vi "Draw GUI running average centroid overlay.vi"(8 "error in":errorcluster, 10 "GUI_centroid overlay":T2={"CentroidX array"=[], "CentroidY array"=[], "CentroidX"=0.0, "CentroidY"=0.0, "# images to average"=1250067, "Overlay Size"={"xhair size"=0.0, "xhair size 2"=0.0}, "Color"=1250067, "Draw"=FALSE, "Thickness"=0}, 11 "Image in":T3) -> (0 "error out":errorcluster, 3 "image out":T3)   [LabVIEW 2020]
doc: "Draw Crosshair in image as per targetx and y and size\ninput:\n1. Draw crosshair cluster (Image in, Draw(boolean), size, target x, target y)\n2. Error in\noutput\n1.Error out"
uses:
  <vilib>/vision/Image Controls.llb/IMAQ Image.ctl
  Controls/GUI_running average centroid overlay.ctl
  General GUIs/Device GUIs/GUI_Cameras/Controls/Crosshair type def.ctl
  <vilib>/ptbypt/NI_PtbyPt.lvlib
panel:
  in  "Crosshair":T1={"Draw"=TRUE, "Target"={"x"=75.0, "y"=100.0}, "Size"={"x"=75.0, "y"=100.0}, "Angle"=1250067.0, "Color"=1250067, "Thickness"=20, "CrosshairLabel"=""} {"Thickness" max=0; "Angle" format="%#_13g"; "Size"."y" min=0.0 max=0.0; "Size"."x" min=0.0 max=0.0}
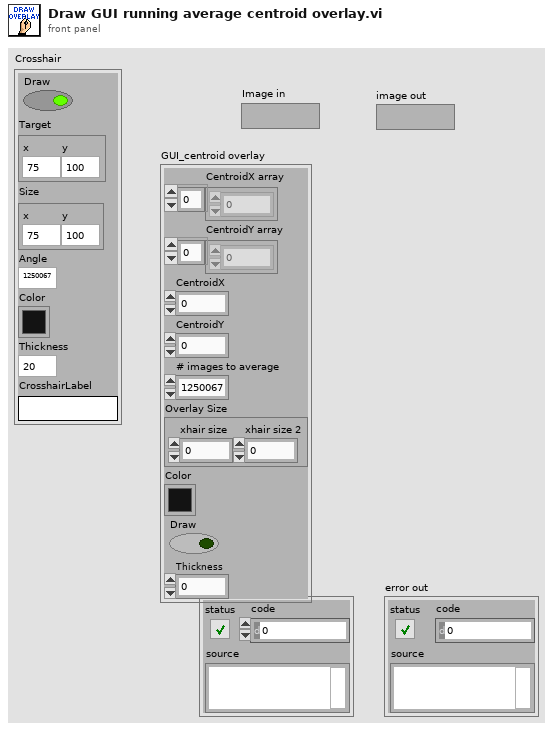
[diagram p1: front panel]
types:
  T1 = typedef "Crosshair type def.ctl" = cluster{"Draw":bool, "Target":cluster{"x":dbl, "y":dbl}, "Size":cluster{"x":dbl, "y":dbl}, "Angle":dbl, "Color":u32, "Thickness":u8, "CrosshairLabel":string}
  T2 = typedef "GUI_running average centroid overlay.ctl" = cluster{"CentroidX array":dbl[], "CentroidY array":dbl[], "CentroidX":dbl, "CentroidY":dbl, "# images to average":i32, "Overlay Size":cluster{"xhair size":dbl, "xhair size 2":dbl}, "Color":u32, "Draw":bool, "Thickness":u8}
  T3 = typedef "IMAQ Image.ctl" = refnum<image>
  T4 = cluster{"Left":i32, "Top":i32, "Right":i32, "Bottom":i32}
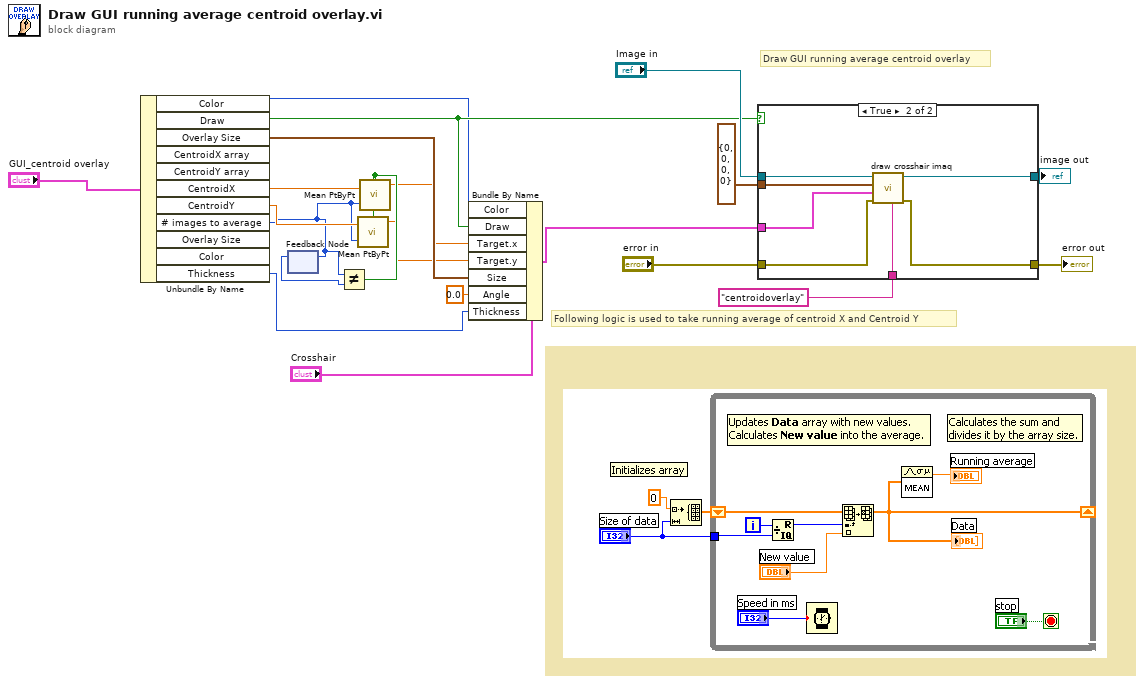
[diagram p0: block diagram]
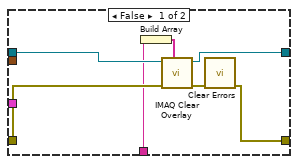
[diagram p2: hidden frame]
diagram:
  # "Following logic is used to take running average of centroid X and Centroid Y"
  # "Draw GUI running average centroid overlay"
  n1 = Unbundle By Name("GUI_centroid overlay") -> ("Color"=w3:u32, "Draw"=w7:bool, "Overlay Size"=w6:cluster{"xhair size":dbl, "xhair size 2":dbl}, "CentroidX"=w14:dbl, "CentroidY"=w13:dbl, "# images to average"=w12:i32, "Thickness"=w1:u8)  [unwired: 4 out]
  n2 = feedback-in #1(w12) -> ()
  n3 = feedback #1() -> (w11:i32)  [unwired: 1 in]
  n4 = Not Equal?(x=w12, y=w11) -> (x != y?=w10:bool)
  n5 = call <vilib>:"Mean PtByPt.vi"("x"=w13, "sample length"=w12, "initialize"=w10) -> ("mean"=w4:dbl)  [unwired: 1 in, 1 out]
  n6 = call <vilib>:"Mean PtByPt.vi"("x"=w14, "sample length"=w12, "initialize"=w10) -> ("mean"=w5:dbl)  [unwired: 1 in, 1 out]
  n7 = Bundle By Name(cluster="Crosshair", "Color"=w3, "Draw"=w7, "Target.x"=w5, "Target.y"=w4, "Size"=w6, "Angle"=0.0, "Thickness"=w1) -> (w9:T1)
  n8 = case shown="True" w7 {
    tunnel: w9 -> [_ w29]
    tunnel: "Image in" -> [w28 w35]
    tunnel: [w27 w33] -> w17
    tunnel: T4 {"Left"=0, "Top"=0, "Right"=0, "Bottom"=0} ("Bounding Rectangle") -> [_ w34]
    tunnel: "error in" -> [w26 w32]
    tunnel: [w25 w31] -> w20
    tunnel: "centroidoverlay" ("overlay name") -> [w22 w30]
    frame False {
      n9 = Build Array(w22) -> (w23:string[])
      n10 = call "IMAQ Clear Overlay"("Groups"=w23, "error in (no error)"=w26, "Image"=w28) -> ("error out"=w24:errorcluster, "Image Out"=w27:T3)  [unwired: 7 in]
      n11 = call <vilib>:"Clear Errors.vi"("error in (no error)"=w24) -> ("error out"=w25:errorcluster)  [unwired: 5 in, 1 out]
    }
    frame True {
      n12 = call "draw crosshair imaq.vi"("overlay name"=w30, "error in (no error)"=w32, "Crosshair"=w29, "Bounding Rectangle"=w34, "image in"=w35) -> ("error out"=w31:errorcluster, "image out"=w33:T3)  [unwired: 5 in]
    }
  }
  "error out" <- w20
  "image out" <- w17
